vi "Current Nominal Write Array.vi"(8 "error in":errorcluster, 10 "Current Nominal AV":dbl[](array[numeric]), 11 "Cycler in":refnum<class "Cycler.lvclass">) -> (0 "error out":errorcluster, 3 "Cycler out":refnum<class "Cycler.lvclass">)   [LabVIEW 2023, in "Cycler.lvclass"]
uses:
  Cycler.lvclass
  Cycler.lvclass/Cycler.ctl
  Low Level Capabilities/Current/Current Nominal Value/Current Nominal Value.lvclass
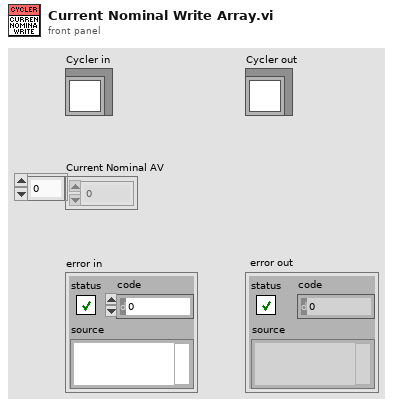
[diagram p1: front panel]
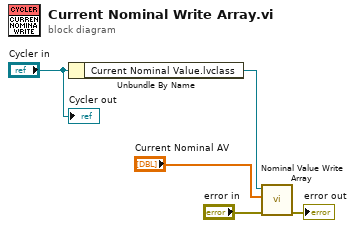
[diagram p0: block diagram]
diagram:
  n1 = Unbundle By Name("Cycler in") -> ("Current Nominal Value.lvclass"=w4:refnum<class "Current Nominal Value.lvclass">)
  n2 = call-dynamic "Nominal Value Write Array.vi"("Current Nominal Value in"=w4, "Current Nominal Value Value"="Current Nominal AV", "error in"="error in") -> ("error out"=→"error out":errorcluster)  [unwired: 6 in, 1 out]
  "Cycler out" <- "Cycler in"
